vi "Show Panel.vi"(8 "error in (no error)":errorcluster) -> (0 "error out":errorcluster)   [LabVIEW 2015, in "Tool Module.lvlib"]
doc: "Send the Show Panel request to the Module's Main.vi.\n_____\nBased on Delacor QMH Project Template 2.1.0.2."
uses:
  Tool Module.lvlib
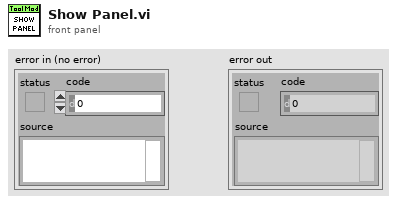
[diagram p1: front panel]
types:
  T1 = typedef "Tool Module.lvlib/Request Events--cluster.ctl" = cluster{"Stop Module":refnum<user-event>, "Show Panel":refnum<user-event>, "Hide Panel":refnum<user-event>, "Get Module Execution Status":refnum<user-event>, "Show Diagram":refnum<user-event>, "Test Trig 2":refnum<user-event>, "GOTO":refnum<user-event>, "Start Inspect":refnum<user-event>, "CONNECT":refnum<user-event>, "Get All Inspect Data":refnum<user-event>, "Get Inspection Limits":refnum<user-event>, "Set Inspection Limits":refnum<user-event>, "Update Status":refnum<user-event>, "Start Data Monitor":refnum<user-event>, "Get FPGA Setup Params":refnum<user-event>, "Set FPGA Setup Params":refnum<user-event>, "Set Tool Config":refnum<user-event>, "Get Tool Config":refnum<user-event>, "Set Integration Count":refnum<user-event>, "Set Laser Params":refnum<user-event>, "Get Mtrl Ctrl Reg":refnum<user-event>, "Commit Ctrl Reg":refnum<user-event>, "Set Event Logger":refnum<user-event>, "Write to File":refnum<user-event>, "Read from File":refnum<user-event>, "Set Device Temp Thresholds":refnum<user-event>, "Get Cycle Count":refnum<user-event>}
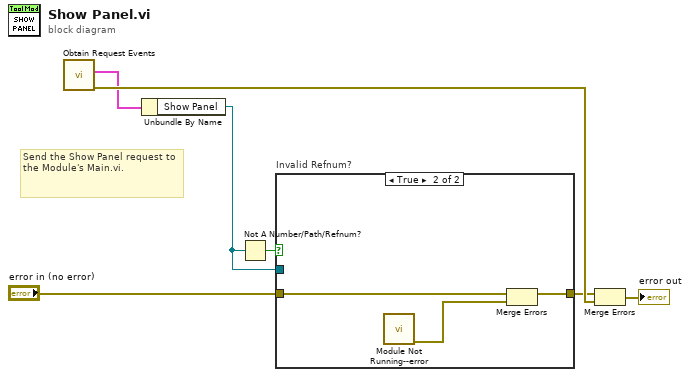
[diagram p0: block diagram]
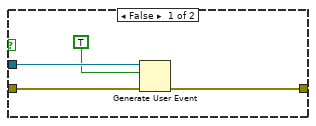
[diagram p2: hidden frame]
diagram:
  # "Send the Show Panel request to the Module's Main.vi."
  n1 = call "Obtain Request Events.vi"() -> ("error out"=w6:errorcluster, "Tool Module Request Events"=w5:T1)  [unwired: 10 in]
  n2 = Unbundle By Name(w5) -> ("Show Panel"=w3:refnum<user-event>)
  n3 = Not A Number/Path/Refnum?(number/path/refnum=w3) -> (NaN/Path/Refnum?=w4:bool)
  n4 = case "Invalid Refnum?" shown="True" w4 {
    tunnel: "error in (no error)" -> [w11 w14]
    tunnel: [w10 w13] -> w1
    tunnel: w3 -> [w9 _]
    frame False {
      n5 = Generate User Event(user event=w9, event data cluster=TRUE ("event data"), error in=w11) -> (error out=w10:errorcluster)  [unwired: 1 in, 1 out]
    }
    frame True {
      n6 = call "Module Not Running--error.vi"() -> ("error out"=w12:errorcluster)  [unwired: 11 in]
      n7 = Merge Errors(w14, w12) -> (w13:errorcluster)
    }
  }
  n8 = Merge Errors(w1, w6) -> (→"error out":errorcluster)
